vi "For loop.vi"() -> ()   [LabVIEW 2012]
panel:
  out "Waveform Graph":cluster{dbl, dbl, dbl[]}(graph)
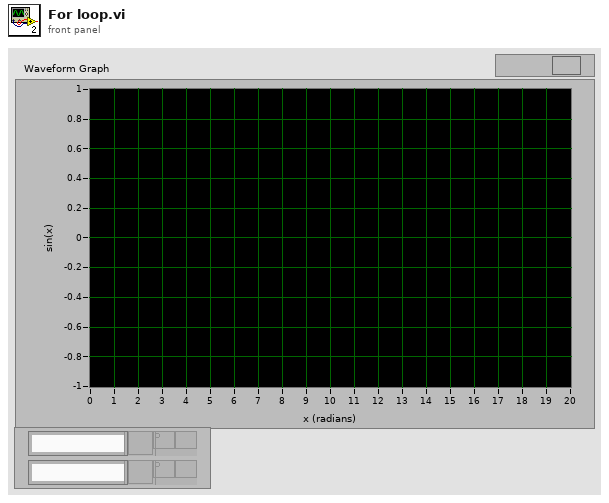
[diagram p1: front panel]
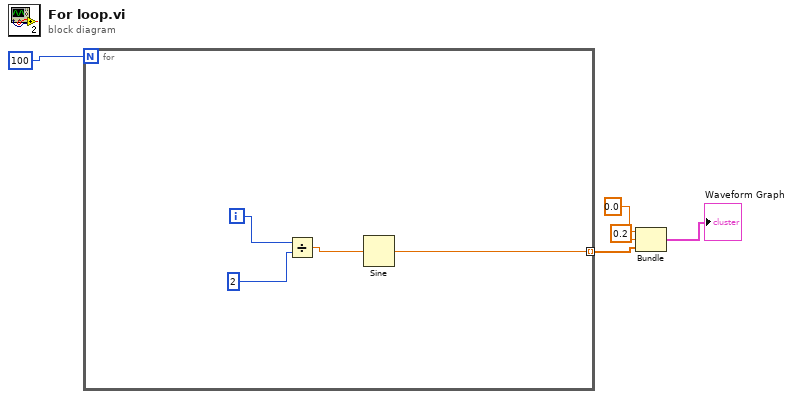
[diagram p0: block diagram]
diagram:
  n1 = for {
    N: 100 -> [_]
    tunnel: [w6] -> w2 mode=indexing
    i -> [w9]
    n2 = Divide(x=w9, y=2) -> (x/y=w7:dbl)
    n3 = Sine(x=w7) -> (sin(x)=w6:dbl)
  }
  n4 = Bundle(0.0, 0.2, w2) -> (→"Waveform Graph":cluster{dbl, dbl, dbl[]})  [unwired: 1 in]
